vi "UM.vi"() -> ()   [LabVIEW 2020]
uses:
  Machine.ctl
  Arrays.ctl
  Array.ctl
  Platter.ctl
panel:
  out "instruction":T1 format="%032b"
  out "Numeric":i32
  in  "wait":u16(slide)=10 max=1000 scale=0.0..1000.0
  out "V":T1 format="%032b"
  out "O":i32
  in  "OK Button":bool
  in  "Path":path=path "/Users/toshi/Documents/UM/codex.umz"
  out "output":string
  out "current machine":T2={"Arrays"={}, "Finger"=0, "Registers"=[], "next id"=1} {"Registers" format="%032b"; "Arrays"."Array" format="%032b"}
  in  "input":string="(\\b.bb)(\\v.vv)06FHPVboundvarHRAk"
  in  "initial array of 2,3":u32[](array[numeric])=[2684354566, 2684354565, 3489660976, 2684354560] format="%032b"
  out "C":i32
  out "B":i32
  out "A":i32
  out "Platter":T1=268435539 format="%032b"
  out "read program":T4 format="%032b"
  in  "initial program in byte array":u8[](array[numeric])=[0, 0, 0, 83, 16, 0, 0, 83, 32, 0, 0, 151, 80, 0, 0, 10, 176, 0, 0, 4, 160, 0, 0, 4, 176, 0, 0, 4, 160, 0, 0, 4, 208, 0, 0, 48, 160, 0, 0, 0, 208, 0, 0, 0, 192, 0, 0, 24] format="%08b"
  in  "initial machine state":T2={"Arrays"={}, "Finger"=0, "Registers"=[0, 0, 0, 0, 0, 0, 0, 0], "next id"=1} {"Registers" format="%032b"; "Arrays"."Array" format="%032b"}
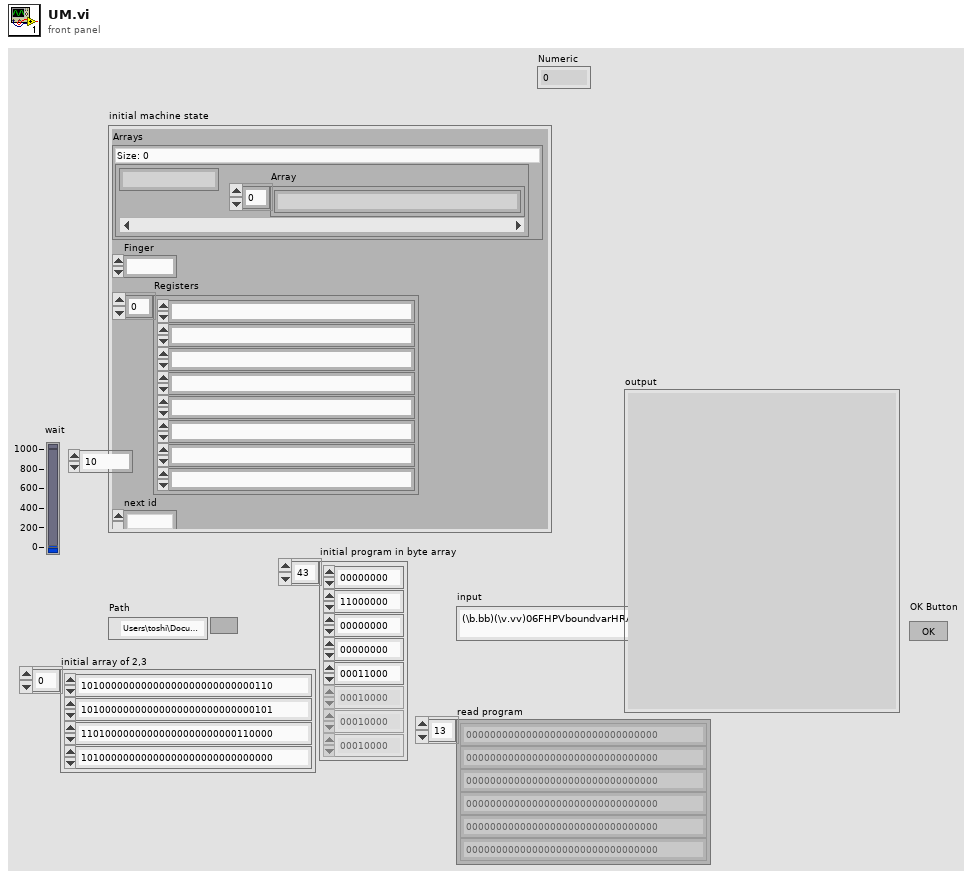
[diagram p1: front panel]
types:
  T1 = typedef "Platter.ctl" = u32
  T2 = typedef "Machine.ctl" = cluster{"Arrays":T3, "Finger":u32, "Registers":T1[], "next id":u32}
  T3 = typedef "Arrays.ctl" = map{string, T4}
  T4 = typedef "Array.ctl" = T1[]
  T5 = enum16{"big-endian, network order", "native, host order", "little-endian"}
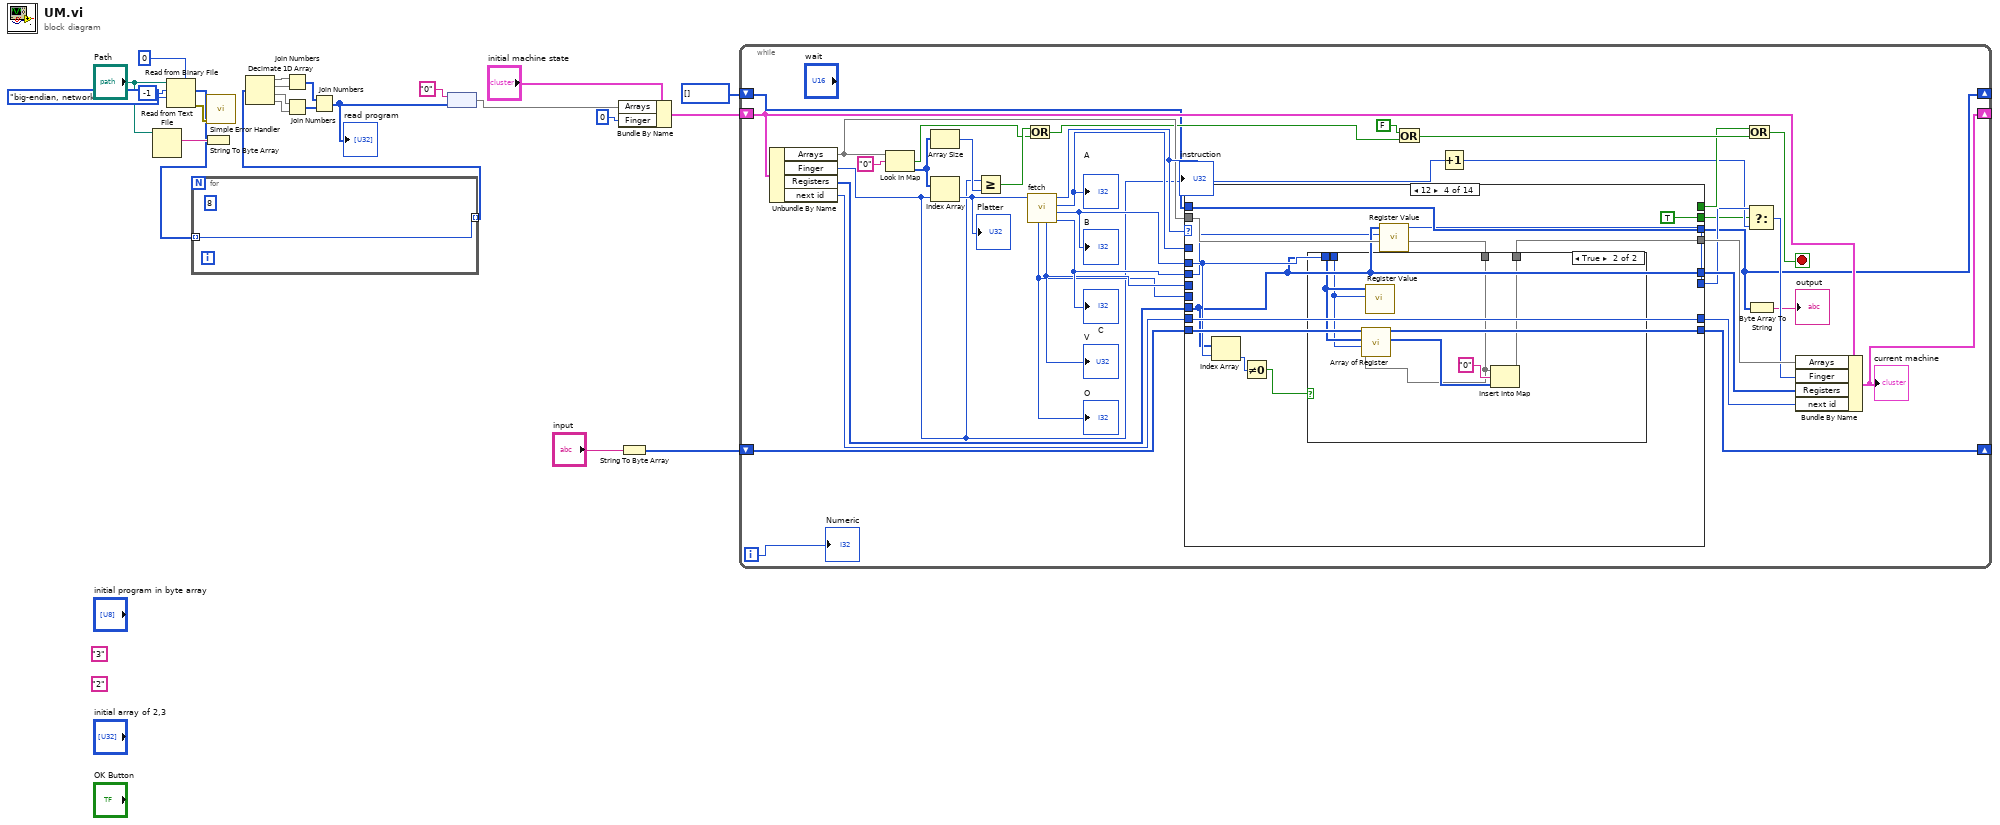
[diagram p0: block diagram]
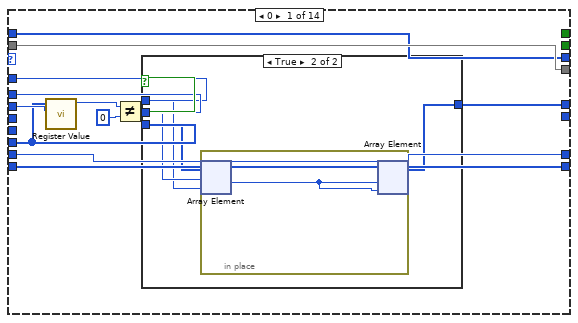
[diagram p2: hidden frame]
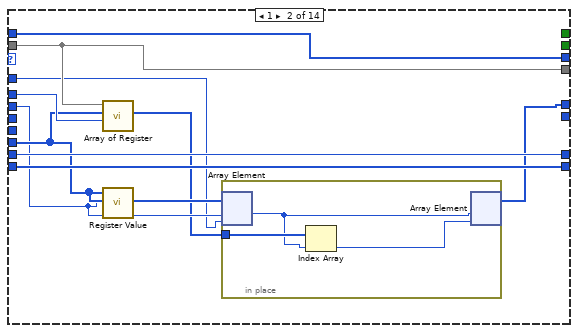
[diagram p4: hidden frame]
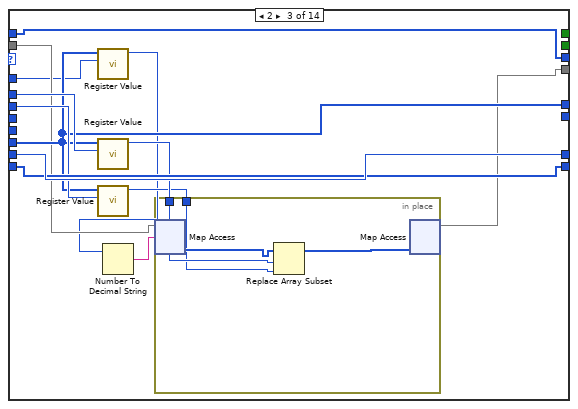
[diagram p5: hidden frame]
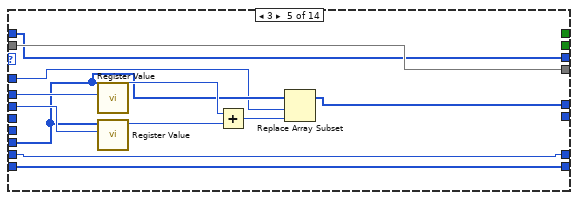
[diagram p7: hidden frame]
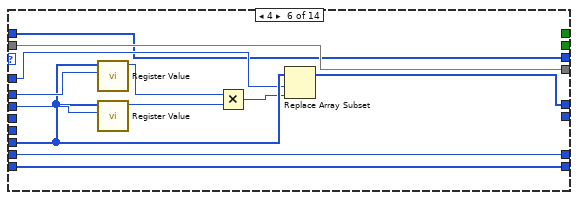
[diagram p8: hidden frame]
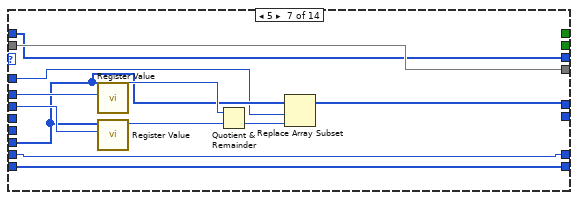
[diagram p9: hidden frame]
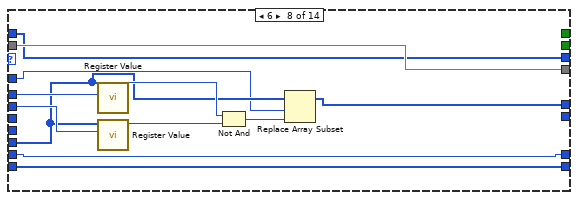
[diagram p10: hidden frame]
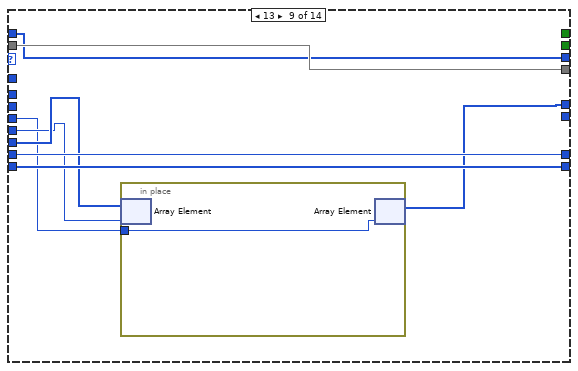
[diagram p11: hidden frame]
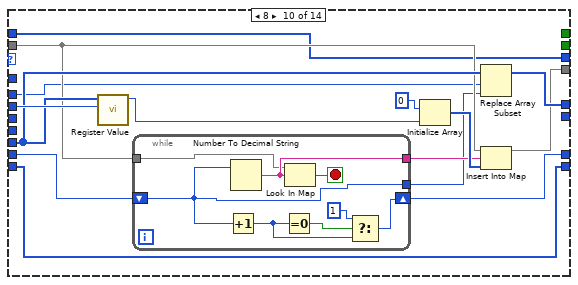
[diagram p12: hidden frame]
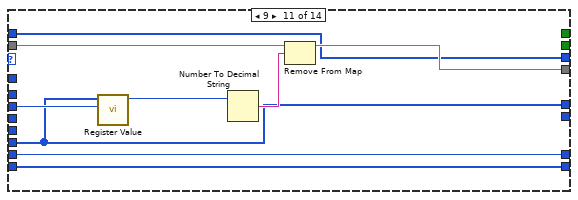
[diagram p13: hidden frame]
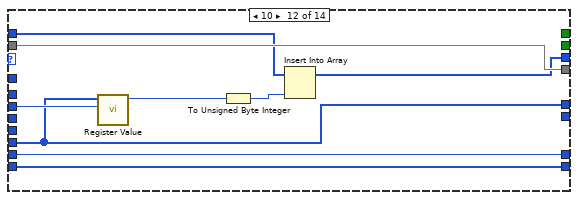
[diagram p14: hidden frame]
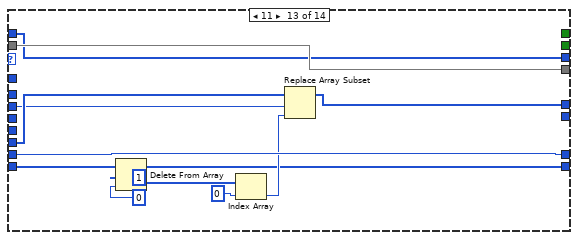
[diagram p15: hidden frame]
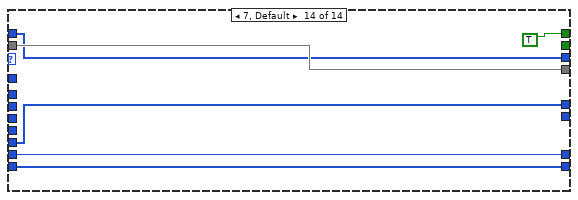
[diagram p16: hidden frame]
diagram:
  (unwired) "3" ("key")
  (unwired) "2" ("key")
  n1 = Read from Text File(file (use dialog)="Path") -> (text=w6:string)  [unwired: 3 in, 3 out]
  n2 = Read from Binary File(5:u8 0, 9:T5."big-endian, network order" ("byte order (0:big-endian, network order)"), 10:-1 ("count (1)"), 11:"Path") -> (0:w8:errorcluster, 2:w3:u8[])  [unwired: 2 in, 2 out]
  n3 = for {
    tunnel: w3 -> [w24] mode=indexing
    tunnel: [w24] -> w2 mode=indexing
    (unwired) 8
  }
  n4 = String To Byte Array(string=w6) -> ()  [unwired: 1 out]
  n5 = call <vilib>:"Simple Error Handler.vi"("error in (no error)"=w8) -> ()  [unwired: 4 in, 5 out]
  n6 = Decimate 1D Array(w2) -> (w18:u8[], w19:u8[], w20:u8[], w21:u8[])
  n7 = Join Numbers(hi=w18, lo=w19) -> ((hi.lo)=w22:u16[])
  n8 = Join Numbers(hi=w20, lo=w21) -> ((hi.lo)=w23:u16[])
  n9 = Join Numbers(hi=w22, lo=w23) -> ((hi.lo)=w16:u32[])
  "read program" <- w16
  n10 = node("0" ("key"), w16) -> (w15:map{string, u32[]})
  n11 = Bundle By Name(cluster="initial machine state", "Arrays"=w15, "Finger"=u32 0) -> (w12:T2)
  n12 = String To Byte Array(string="input") -> (unsigned byte array=w9:u8[])
  n13 = while {
    shift-right: [w52] -> _
    shift-left: w12 -> [w53]
    shift-right: [w28] -> _
    shift-left: u8[] [] -> [w38]
    shift-right: [w36] -> _
    shift-left: w9 -> [w37]
    i -> [w25]
    stop <- w42 stop-if-true
    n14 = Unbundle By Name(w53) -> ("Arrays"=w51:T3, "Finger"=w26:u32, "Registers"=w55:T1[], "next id"=w40:u32)
    n15 = Look In Map(map=w51, key="0") -> (key not found?=w44:bool, value=w47:T4)  [unwired: 1 in]
    n16 = Array Size(array=w47) -> (size(s)=w46:i32)
    n17 = Index Array(array=w47, index=w26) -> (element=w27:T1)
    "Platter" <- w27
    n18 = Greater Or Equal?(x=w26, y=w46) -> (x >= y?=w45:bool)
    n19 = Or(x=w45, y=w44) -> (x .or. y?=w43:bool)
    n20 = call "fetch.vi"("Platter in"=w27) -> ("C"=w57:i32, "B"=w58:i32, "A"=w59:i32, "instruction"=w60:T1, "V"=w31:T1, "O"=w30:i32)  [unwired: 5 in]
    "A" <- w59
    "B" <- w58
    "C" <- w57
    "O" <- w30
    "V" <- w31
    "instruction" <- w60
    n21 = case shown="12" w60 {
      tunnel: w59 -> [w69 w81 w96 _ w133 w145 w157 w169 _ _ _ _ _ _]
      tunnel: w58 -> [w70 w88 w101 w113 w139 w151 w163 w175 _ w187 _ _ _ _]
      tunnel: w57 -> [w63 w82 w100 w110 w138 w150 w162 w174 _ w199 w216 w225 w234 _]
      tunnel: w55 -> [w62 w83 w99 w112 w134 w146 w158 w170 w179 w198 w210 w223 w235 w243]
      tunnel: [w68 w79 w99 w112 w131 w143 w155 w167 w176 w197 w210 w223 w227 w243] -> w54
      tunnel: [w67 w84 w93 w111 w137 w149 w161 w173 w183 w191 w211 w222 w237 w244] -> w50
      tunnel: w51 -> [w67 w84 w98 w114 w137 w149 w161 w173 w183 w189 w212 w222 w237 w244]
      tunnel: [_ _ _ _ _ _ _ _ _ _ _ _ _ TRUE ("x")] -> w41
      tunnel: w40 -> [w66 w87 w104 w120 w130 w142 w154 w166 w182 w196 w215 w224 w238 w241]
      tunnel: [w66 w87 w104 w120 w130 w142 w154 w166 w182 w195 w215 w224 w238 w241] -> w39
      tunnel: w38 -> [w65 w86 w103 w119 w129 w141 w153 w165 w181 w186 w209 w219 w236 w240]
      tunnel: [w65 w86 w103 w119 w129 w141 w153 w165 w181 w186 w209 w218 w236 w240] -> w28
      tunnel: w37 -> [w64 w85 w102 w118 w128 w140 w152 w164 w180 w185 w208 w217 w233 w239]
      tunnel: [w64 w85 w102 w118 w128 w140 w152 w164 w180 w185 w208 w217 w226 w239] -> w36
      tunnel: [_ _ _ w109 _ _ _ _ _ _ _ _ _ _] -> w35
      tunnel: [_ _ _ TRUE _ _ _ _ _ _ _ _ _ _] -> w33
      tunnel: w31 -> [_ _ _ _ _ _ _ _ w177 _ _ _ _ _]
      tunnel: w30 -> [_ _ _ _ _ _ _ _ w178 _ _ _ _ _]
      frame 0 {
        n22 = call "Register Value.vi"("Register"=w63, "Registers"=w62) -> ("Platter"=w61:T1)  [unwired: 9 in]
        n23 = Not Equal?(x=w61, y=u32 0) -> (x != y?=w71:bool)
        n24 = case shown="True" w71 {
          tunnel: w62 -> [w73 w77]
          tunnel: w70 -> [_ w76]
          tunnel: w69 -> [_ w75]
          tunnel: [w73 w74] -> w68
          frame False {
          }
          frame True {
            n25 = in-place {
              n26 = in-place-array #1(w77, w76, w75) -> (w78:T1)  [unwired: 1 out]
              n27 = in-place-array #1(w78, w78) -> (w74:T1[])  [unwired: 2 out]
            }
          }
        }
      }
      frame 1 {
        n28 = call "Array of Register.vi"("Register"=w88, "Registers"=w83, "Arrays"=w84) -> ("Array"=w80:T4)  [unwired: 7 in]
        n29 = call "Register Value.vi"("Register"=w82, "Registers"=w83) -> ()  [unwired: 9 in, 1 out]
        n30 = in-place {
          in-place-border: w80 -> [w91]
          n31 = in-place-array #2(w83, w82, w81) -> (w90:T1)  [unwired: 1 out]
          n32 = Index Array(array=w91, index=w90) -> (element=w89:T1)
          n33 = in-place-array #2(w90, w89) -> (w79:T1[])  [unwired: 2 out]
        }
      }
      frame 2 {
        n34 = call "Register Value.vi"("Register"=w96, "Registers"=w99) -> ("Platter"=w92:T1)  [unwired: 9 in]
        n35 = call "Register Value.vi"("Register"=w101, "Registers"=w99) -> ("Platter"=w95:T1)  [unwired: 9 in]
        n36 = call "Register Value.vi"("Register"=w100, "Registers"=w99) -> ("Platter"=w94:T1)  [unwired: 9 in]
        n37 = Number To Decimal String(number=w92) -> (decimal integer string=w97:string)  [unwired: 1 in]
        n38 = in-place {
          in-place-border: w95 -> [w107]
          in-place-border: w94 -> [w106]
          n39 = in-place-map #3(w98, w97) -> (w108:T4)  [unwired: 1 in, 1 out]
          n40 = Replace Array Subset(array=w108, new element=w106, index=w107) -> (w105:T4)
          n41 = in-place-map #3(w105) -> (w93:T3)  [unwired: 1 in, 2 out]
        }
      }
      frame 12 {
        n42 = Index Array(array=w112, index=w113) -> (element=w115:T1)
        n43 = Not Equal To 0?(x=w115) -> (x != 0?=w116:bool)
        n44 = case shown="True" w116 {
          tunnel: w114 -> [w121 w125]
          tunnel: w113 -> [_ w122]
          tunnel: w112 -> [_ w123]
          tunnel: [w121 w124] -> w111
          frame False {
          }
          frame True {
            n45 = call "Array of Register.vi"("Register"=w122, "Registers"=w123, "Arrays"=w125) -> ("Array"=w127:T4)  [unwired: 7 in]
            n46 = call "Register Value.vi"("Register"=w122, "Registers"=w123) -> ()  [unwired: 9 in, 1 out]
            n47 = Insert Into Map(map in=w125, key="0", value=w127) -> (map out=w124:T3)  [unwired: 2 out]
          }
        }
        n48 = call "Register Value.vi"("Register"=w110, "Registers"=w112) -> ("Platter"=w109:T1)  [unwired: 9 in]
      }
      frame 3 {
        n49 = call "Register Value.vi"("Register"=w139, "Registers"=w134) -> ("Platter"=w136:T1)  [unwired: 9 in]
        n50 = call "Register Value.vi"("Register"=w138, "Registers"=w134) -> ("Platter"=w135:T1)  [unwired: 9 in]
        n51 = Add(x=w136, y=w135) -> (x+y=w132:T1)
        n52 = Replace Array Subset(array=w134, new element=w132, index=w133) -> (w131:T1[])
      }
      frame 4 {
        n53 = call "Register Value.vi"("Register"=w151, "Registers"=w146) -> ("Platter"=w148:T1)  [unwired: 9 in]
        n54 = call "Register Value.vi"("Register"=w150, "Registers"=w146) -> ("Platter"=w147:T1)  [unwired: 9 in]
        n55 = Multiply(x=w148, y=w147) -> (x*y=w144:T1)
        n56 = Replace Array Subset(array=w146, new element=w144, index=w145) -> (w143:T1[])
      }
      frame 5 {
        n57 = call "Register Value.vi"("Register"=w163, "Registers"=w158) -> ("Platter"=w160:T1)  [unwired: 9 in]
        n58 = call "Register Value.vi"("Register"=w162, "Registers"=w158) -> ("Platter"=w159:T1)  [unwired: 9 in]
        n59 = Quotient & Remainder(x=w160, y=w159) -> (floor(x/y)=w156:T1)  [unwired: 1 out]
        n60 = Replace Array Subset(array=w158, new element=w156, index=w157) -> (w155:T1[])
      }
      frame 6 {
        n61 = call "Register Value.vi"("Register"=w175, "Registers"=w170) -> ("Platter"=w172:T1)  [unwired: 9 in]
        n62 = call "Register Value.vi"("Register"=w174, "Registers"=w170) -> ("Platter"=w171:T1)  [unwired: 9 in]
        n63 = Not And(1:w171, 2:w172) -> (0:w168:T1)
        n64 = Replace Array Subset(array=w170, new element=w168, index=w169) -> (w167:T1[])
      }
      frame 13 {
        n65 = in-place {
          in-place-border: w177 -> [w184]
          n66 = in-place-array #4(w179, w178) -> ()  [unwired: 1 out]
          n67 = in-place-array #4(w184) -> (w176:T1[])  [unwired: 1 out]
        }
      }
      frame 8 {
        n68 = call "Register Value.vi"("Register"=w199, "Registers"=w198) -> ("Platter"=w194:T1)  [unwired: 9 in]
        n69 = while {
          shift-right: [w205] -> w195
          shift-left: w196 -> [w201]
          tunnel: [w202] -> w192
          tunnel: [w201] -> w188
          tunnel: w189 -> [w200]
          stop <- w207 stop-if-true
          n70 = Increment(x=w201) -> (x+1=w204:u32)
          n71 = Number To Decimal String(number=w201) -> (decimal integer string=w202:string)  [unwired: 1 in]
          n72 = Equal To 0?(x=w204) -> (x = 0?=w206:bool)
          n73 = Look In Map(map=w200, key=w202) -> (key not found?=w207:bool)  [unwired: 1 in, 1 out]
          n74 = Select(t=u32 1, s=w206, f=w204) -> (s? t:f=w205:u32)
        }
        n75 = Initialize Array(T1 0 ("Platter"), w194) -> (w193:T1[])
        n76 = Replace Array Subset(array=w198, new element=w188, index=w187) -> (w197:T1[])
        n77 = Insert Into Map(map in=w189, key=w192, value=w193) -> (map out=w191:T3)  [unwired: 2 out]
      }
      frame 9 {
        n78 = call "Register Value.vi"("Register"=w216, "Registers"=w210) -> ("Platter"=w213:T1)  [unwired: 9 in]
        n79 = Number To Decimal String(number=w213) -> (decimal integer string=w214:string)  [unwired: 1 in]
        n80 = Remove From Map(10:w214, 11:w212) -> (3:w211:T3)  [unwired: 2 out]
      }
      frame 10 {
        n81 = call "Register Value.vi"("Register"=w225, "Registers"=w223) -> ("Platter"=w221:T1)  [unwired: 9 in]
        n82 = To Unsigned Byte Integer(number=w221) -> (unsigned 8bit integer=w220:u8)
        n83 = Insert Into Array(array=w219, new element=w220) -> (w218:u8[])  [unwired: 1 in]
      }
      frame 11 {
        n84 = Delete From Array(array=w233, length=1, index=0) -> (deleted portion=w230:u8[], array with subset deleted=w226:u8[])
        n85 = Index Array(array=w230, index=0) -> (element=w228:u8)
        n86 = Replace Array Subset(array=w235, new element=w228, index=w234) -> (w227:T1[])
      }
      frame 7, Default {
      }
    }
    n87 = Or(x=FALSE, y=w43) -> (x .or. y?=w48:bool)
    n88 = Increment(x=w26) -> (x+1=w34:u32)
    n89 = Or(x=w41, y=w48) -> (x .or. y?=w42:bool)
    n90 = Select(t=w35, s=w33, f=w34) -> (s? t:f=w32:T1)
    n91 = Byte Array To String(unsigned byte array=w28) -> (string=→"output":string)
    n92 = Bundle By Name(cluster=w53, "Arrays"=w50, "Finger"=w32, "Registers"=w54, "next id"=w39) -> (w52:T2)
    "current machine" <- w52
    "Numeric" <- w25
  }
